vi "Multidimensional Arrays.vi"() -> ()   [LabVIEW 2019]
panel:
  out "transposed array":dbl[][](array[numeric])
  in  "Array":dbl[][](array[numeric])
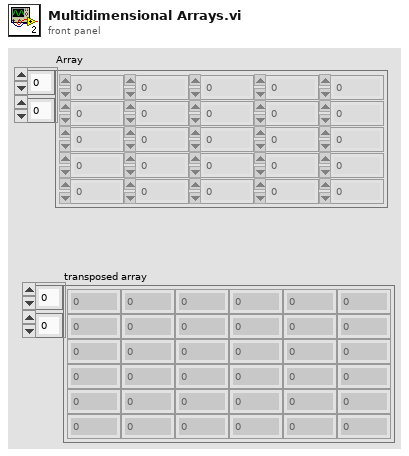
[diagram p1: front panel]
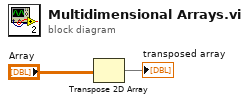
[diagram p0: block diagram]
diagram:
  n1 = Transpose 2D Array(2D array="Array") -> (transposed array=→"transposed array":dbl[][])
